vi "G4BaseTemplate_Simple_4x4x4_GetAttributes.vi"(8 "error in (no error)":errorcluster, 10 "OnlyGetDvrReference(False)":bool, 11 "reference in":refnum<class "G4BaseTemplate_Simple_4x4x4.lvclass">) -> (0 "error out":errorcluster, 1 "DataRef":refnum<data-value>, 2 "Data":T1 {"Attribute1" format="%.2f"}, 3 "reference out":refnum<class "G4BaseTemplate_Simple_4x4x4.lvclass">)   [LabVIEW 2014, in "G4BaseTemplate_Simple_4x4x4.lvclass"]
uses:
  <resource>/Framework/Providers/Open_GDS/ClassProviders/Provider_EndevoGOOP400/Templates/G4BaseTemplate_Simple_4x4x4/G4BaseTemplate_Simple_4x4x4.lvclass
  <resource>/Framework/Providers/Open_GDS/ClassProviders/Provider_EndevoGOOP400/Templates/G4BaseTemplate_Simple_4x4x4/protected/ObjectAttributes.ctl
  <resource>/Framework/Providers/Open_GDS/ClassProviders/Provider_EndevoGOOP400/Templates/G4BaseTemplate_Simple_4x4x4/G4BaseTemplate_Simple_4x4x4.lvclass/G4BaseTemplate_Simple_4x4x4.ctl
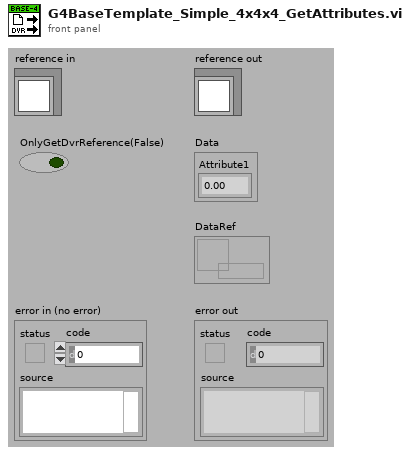
[diagram p1: front panel]
types:
  T1 = typedef "G4BaseTemplate_Simple_4x4x4.lvclass/ObjectAttributes.ctl" = cluster{"Attribute1":dbl}
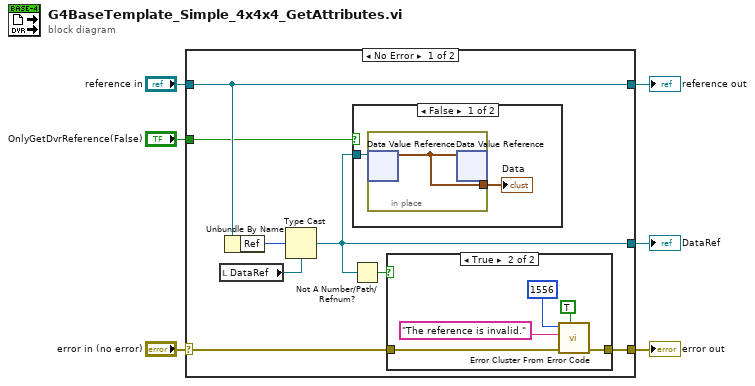
[diagram p0: block diagram]
diagram:
  n1 = case shown="No Error" "error in (no error)" {
    selector: "error in (no error)" -> [w8 w24]
    tunnel: [w7 w24] -> w5
    tunnel: [w14 w25] -> w3
    tunnel: "reference in" -> [w14 w25]
    tunnel: [w9 _] -> w2
    tunnel: "OnlyGetDvrReference(False)" -> [w11 _]
    frame No Error {
      n2 = local read "DataRef"() -> (w12:refnum<data-value>)
      n3 = Unbundle By Name(w14) -> ("Ref"=w13:u32)
      n4 = Type Cast(type=w12, x=w13) -> (*(type *) &x=w9:refnum<data-value>)
      n5 = Not A Number/Path/Refnum?(number/path/refnum=w9) -> (NaN/Path/Refnum?=w10:bool)
      n6 = case shown="False" w11 {
        tunnel: w9 -> [w22 _]
        frame False {
          n7 = in-place {
            in-place-border: [w23] -> w21
            n8 = in-place-dvr #1(w22) -> (w23:T1)  [unwired: 1 out]
            n9 = in-place-dvr #1(w23) -> ()  [unwired: 2 out]
          }
          "Data" <- w21
        }
        frame True {
        }
      }
      n10 = case shown="True" w10 {
        tunnel: w8 -> [w15 w17]
        tunnel: [w15 w16] -> w7
        frame False {
        }
        frame True {
          n11 = call <vilib>:"Error Cluster From Error Code.vi"("show call chain? (False)"=TRUE, "error in (no error)"=w17, "error message (\"\")"="The reference is invalid." ("source"), "error code (0)"=1556 ("code")) -> ("error out"=w16:errorcluster)  [unwired: 5 in]
        }
      }
    }
    frame Error {
    }
  }
  "error out" <- w5
  "reference out" <- w3
  "DataRef" <- w2
